vi "TestExec.Maintenance Interval Check.vi"(7 "Health":T1, 8 "error in (no error)":errorcluster, 11 "Main Q":refnum<queue>) -> (0 "error out":errorcluster, 3 "Main Q Dup":refnum<queue>)   [LabVIEW 2018]
uses:
  Controls and Type Defs/TestExec.Health Management Params.ctl
  <vilib>/KATE/Queues/Q.Element.ctl
  <vilib>/KATE/Scheduler/Scheduler.lvlib
  <vilib>/KATE/Queues/Queue Utils.lvlib
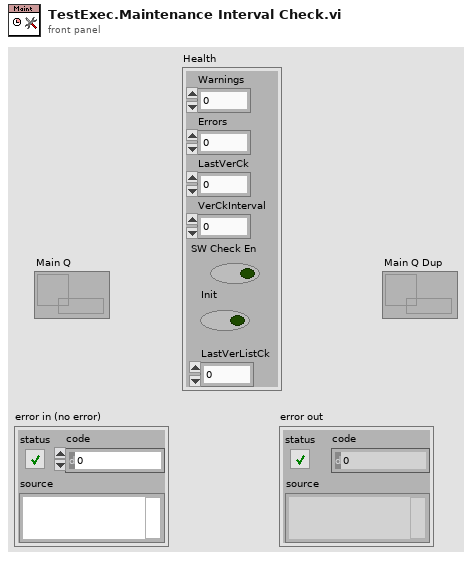
[diagram p1: front panel]
types:
  T1 = typedef "TestExec.Health Management Params.ctl" = cluster{"Warnings":i32, "Errors":i32, "LastVerCk":dbl, "VerCkInterval":dbl, "SW Check En":bool, "Init":bool, "LastVerListCk":dbl}
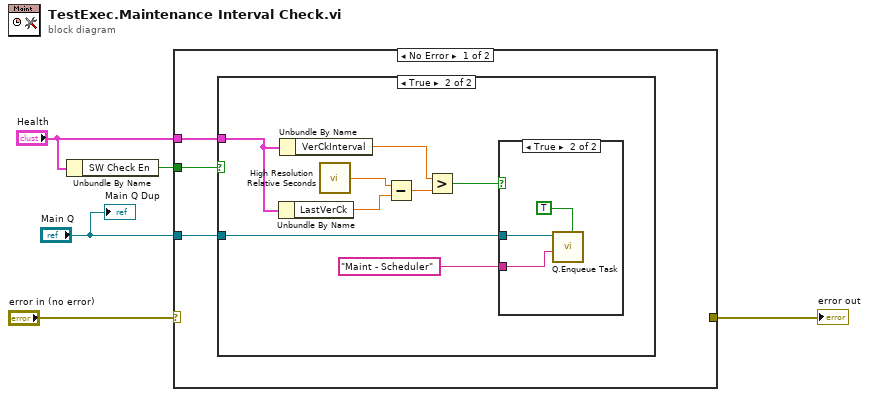
[diagram p0: block diagram]
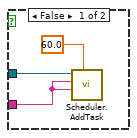
[diagram p3: hidden frame]
diagram:
  n1 = Unbundle By Name("Health") -> ("SW Check En"=w2:bool)
  n2 = case shown="No Error" "error in (no error)" {
    selector: "error in (no error)" -> [_ w23]
    tunnel: [_ w23] -> w4
    tunnel: "Health" -> [w8 _]
    tunnel: w2 -> [w7 _]
    tunnel: "Main Q" -> [w6 _]
    frame No Error {
      n3 = case shown="True" w7 {
        tunnel: w8 -> [_ w11]
        tunnel: w6 -> [_ w9]
        frame False {
        }
        frame True {
          n4 = Unbundle By Name(w11) -> ("LastVerCk"=w16:dbl)
          n5 = Unbundle By Name(w11) -> ("VerCkInterval"=w13:dbl)
          n6 = call <vilib>:"High Resolution Relative Seconds.vi"() -> ("relative seconds"=w15:dbl)
          n7 = Subtract(x=w15, y=w16) -> (x-y=w14:dbl)
          n8 = Greater?(x=w13, y=w14) -> (0:w10:bool)
          n9 = case shown="True" w10 {
            tunnel: "Maint - Scheduler" -> [w19 w22]
            tunnel: w9 -> [w18 w21]
            frame False {
              n10 = call <vilib>:"Scheduler.AddTask.vi"("Interval(s)"=60.0, "Task Name"=w19, "Sched Name"=w19, "Q In"=w18) -> ()  [unwired: 6 in, 2 out]
            }
            frame True {
              n11 = call <vilib>:"Q.Enqueue Task.vi"("Top of Q"=TRUE, "Task Name"=w22, "Q In"=w21) -> ()  [unwired: 7 in, 2 out]
            }
          }
        }
      }
    }
    frame Error {
    }
  }
  "error out" <- w4
  "Main Q Dup" <- "Main Q"
